vi "Resample_PASdata.vi"(8 "error in":errorcluster, 11 "PAS in":refnum<class "PAS.lvclass">) -> (0 "error out":errorcluster, 3 "PAS out":refnum<class "PAS.lvclass">)   [LabVIEW 2016, in "PAS Library.lvlib" / "PAS.lvclass"]
uses:
  Main/PAS.lvclass
  G:/sw_repo/For Builds/Reusable/Instrument/Instrument.lvclass
  PAS Data.lvclass
  G:/sw_repo/For Builds/Reusable/Data/Data.lvclass
  Instrument/Instrument.lvclass/Instrument.ctl
  Instrument/Read Data.vi
  Instrument/Write Data.vi
  Read CellData.vi
  Data/Data.lvclass
  Cell/PAS Cell Data.lvclass
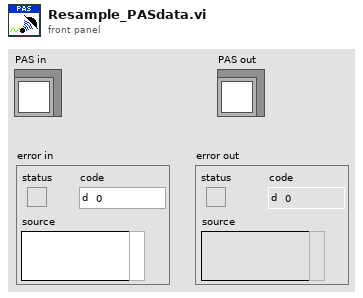
[diagram p1: front panel]
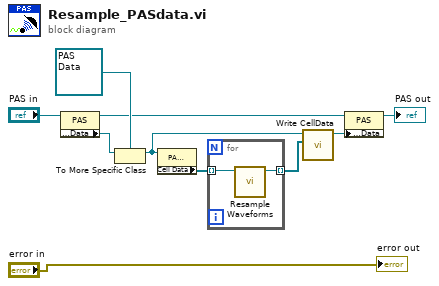
[diagram p0: block diagram]
diagram:
  n1 = property class="PAS"(reference="PAS in") -> (reference out=w3:refnum<class "PAS.lvclass">, "Accessors:Data"=w8:refnum<class "Data.lvclass">)  [unwired: 1 in, 1 out]
  n2 = To More Specific Class(target class=refnum<class "PAS Data.lvclass"> refnum ("reference"), reference=w8) -> (specific class reference=w5:refnum<class "PAS Data.lvclass">)  [unwired: 1 in, 1 out]
  n3 = property class="PAS Data"(reference=w5) -> ("Cell Data"=w7:refnum<class "PAS Cell Data.lvclass">[])  [unwired: 1 in, 2 out]
  n4 = for {
    tunnel: w7 -> [w12] mode=indexing
    tunnel: [w11] -> w6 mode=indexing
    n5 = call "Resample Waveforms.vi"("PAS Cell Data in"=w12) -> ("PAS Cell Data out"=w11:refnum<class "PAS Cell Data.lvclass">)  [unwired: 9 in, 1 out]
  }
  n6 = call "Write CellData.vi"("CellData"=w6, "PAS Data in"=w5) -> ("PAS Data out"=w4:refnum<class "PAS Data.lvclass">)  [unwired: 8 in, 1 out]
  n7 = property class="PAS"(reference=w3, "Accessors:Data"=w4) -> (reference out=→"PAS out":refnum<class "PAS.lvclass">)  [unwired: 1 in, 1 out]
  "error out" <- "error in"
